vi "SampleGetApi.vi"() -> ()   [LabVIEW 2025]
doc: "Created a get api and stores the resultant response in response body string"
uses:
  <vilib>/httpClient/LabVIEWHTTPClient.lvlib
panel:
  out "response body":string
  # "Sample get api"
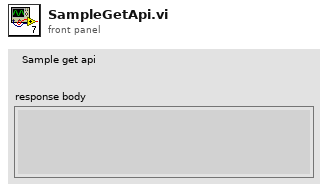
[diagram p1: front panel]
types:
  T1 = typedef "LabVIEWHTTPClient.lvlib/ClientHandle.ctl" = refnum<k1>
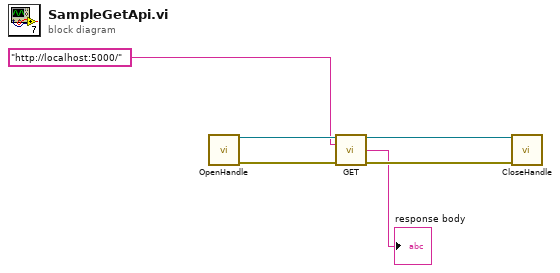
[diagram p0: block diagram]
diagram:
  n1 = call <vilib>:"OpenHandle.vi"() -> ("client handle out"=w5:T1, "error out"=w4:errorcluster)  [unwired: 14 in]
  n2 = call <vilib>:"GET.vi"("client handle"=w5, "url"="http://localhost:5000/", "error in (no error)"=w4) -> ("client handle out"=w6:T1, "body"=→"response body":string, "error out"=w3:errorcluster)  [unwired: 9 in, 1 out]
  n3 = call <vilib>:"CloseHandle.vi"("client handle"=w6, "error in (no error)"=w3) -> ()  [unwired: 13 in, 1 out]
